vi "SysTest-Get Channel Names.vi"(7 "Use channel mapping?":bool, 11 "error in (no error)":errorcluster) -> (4 "AO Names":string[](array[string]), 8 "AI Names":string[](array[string]), 13 "AO Chans":i32[](array[numeric]), 14 "AI Chans":i32[](array[numeric]), 15 "error out":errorcluster)   [LabVIEW 2020]
uses:
  epl-vi-lib/Connection VIs/Type Defs/Output sources.ctl
  epl-vi-lib/Connection VIs/Type Defs/Input sources.ctl
panel:
  in  "Input sources":T1 items=["--unused--", "Probe Mic Right", "Probe Mic Left", "Cal Mic", "ABR", "CAP Right", "CAP Left", "Startle piezo", "Temperature", "Heart rate", "Accelerometer", "Startle piezo 2"]
  in  "Output sources":T2 items=["--unused--", "Right primary", "Right secondary", "Left primary", "Left secondary", "Shocks", "Startle", "Background", "Shaker", "Blue laser"]
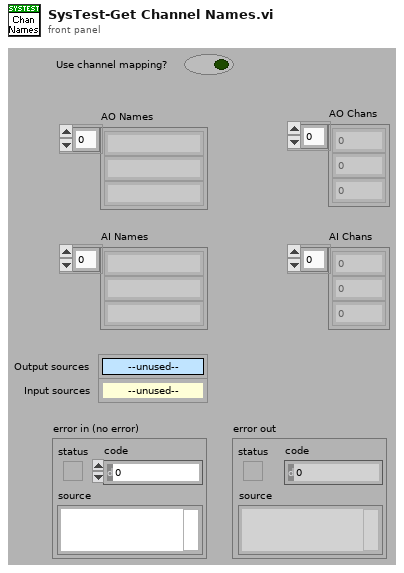
[diagram p1: front panel]
types:
  T1 = typedef "Input sources.ctl" = u16
  T2 = typedef "Output sources.ctl" = u16
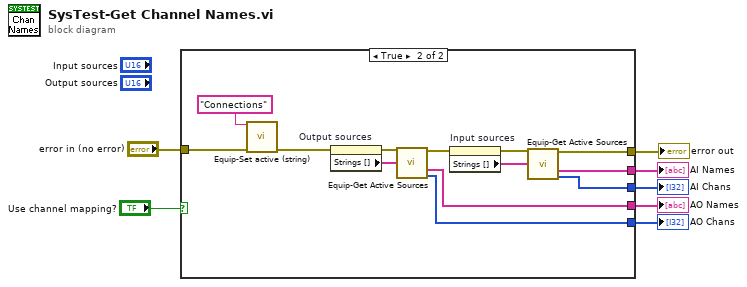
[diagram p0: block diagram]
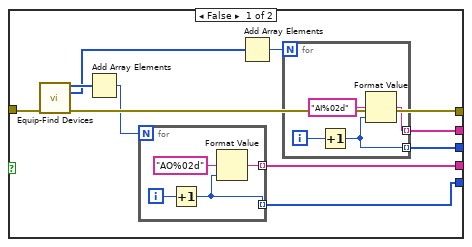
[diagram p2: hidden frame]
diagram:
  n1 = case shown="True" "Use channel mapping?" {
    tunnel: "error in (no error)" -> [w17 w28]
    tunnel: [w9 w33] -> w6
    tunnel: [w8 w32] -> w5
    tunnel: [w12 w31] -> w4
    tunnel: [w13 w30] -> w3
    tunnel: [w15 w29] -> w2
    frame False {
      n2 = call "Equip-Find Devices.vi"("error in (no error)"=w17) -> ("Num AO"=w16:i32[], "Num AI"=w10:i32[], "error out"=w15:errorcluster)  [unwired: 9 in, 3 out]
      n3 = Add Array Elements(numeric array=w16) -> (sum=w14:i32)
      n4 = for {
        N: w14 -> [_]
        tunnel: [w23] -> w13 mode=indexing
        tunnel: [w22] -> w12 mode=indexing
        i -> [w25]
        n5 = Increment(x=w25) -> (x+1=w23:i32)
        n6 = Format Value(format string="AO%02d", value (0)=w23) -> (output string=w22:string)  [unwired: 1 in]
      }
      n7 = Add Array Elements(numeric array=w10) -> (sum=w11:i32)
      n8 = for {
        N: w11 -> [_]
        tunnel: [w19] -> w9 mode=indexing
        tunnel: [w18] -> w8 mode=indexing
        i -> [w20]
        n9 = Increment(x=w20) -> (x+1=w18:i32)
        n10 = Format Value(format string="AI%02d", value (0)=w18) -> (output string=w19:string)  [unwired: 1 in]
      }
    }
    frame True {
      n11 = call "Equip-Set active (string).vi"("Config Name"="Connections", "error in (no error)"=w28) -> ("error out"=w27:errorcluster)  [unwired: 13 in]
      n12 = property on="Output sources" class="Ring (strict)"(error in=w27) -> (error out=w37:errorcluster, "Strings []"=w38:string[])  [unwired: 1 in, 1 out]
      n13 = call "Equip-Get Active Sources.vi"("error in"=w37, "Source Names"=w38) -> ("error out"=w36:errorcluster, "Names"=w31:string[], "Chans"=w30:i32[])  [unwired: 11 in]
      n14 = property on="Input sources" class="Ring (strict)"(error in=w36) -> (error out=w35:errorcluster, "Strings []"=w34:string[])  [unwired: 1 in, 1 out]
      n15 = call "Equip-Get Active Sources.vi"("error in"=w35, "Source Names"=w34) -> ("error out"=w29:errorcluster, "Names"=w33:string[], "Chans"=w32:i32[])  [unwired: 11 in]
    }
  }
  "error out" <- w2
  "AO Names" <- w4
  "AI Names" <- w6
  "AO Chans" <- w3
  "AI Chans" <- w5
